vi "Check motor D2XX.vi"(8 "error in (no error)":errorcluster, 11 "AISAS control in":refnum<class "AISAS motor.lvclass">) -> (0 "error out":errorcluster, 2 "Motor Ok":bool, 3 "AISAS control out":refnum<class "AISAS motor.lvclass">)   [LabVIEW 2014, in "AISAS motor.lvclass"]
uses:
  AISAS motor.lvclass
  Controls/motor.ctl
  AISAS motor.lvclass/AISAS motor.ctl
panel:
  out "Motor":T1
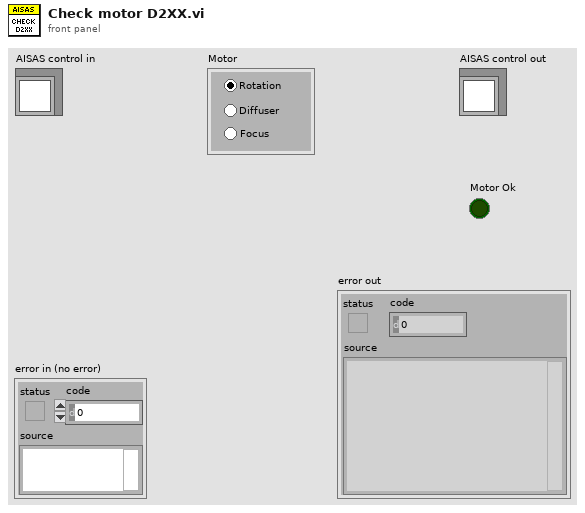
[diagram p1: front panel]
types:
  T1 = typedef "motor.ctl" = enum32{"Rotation", "Diffuser ", "Focus"}
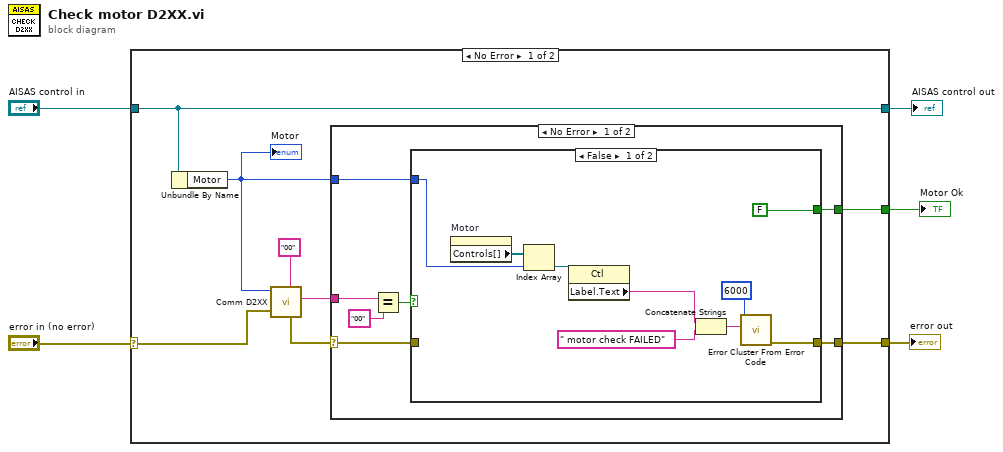
[diagram p0: block diagram]
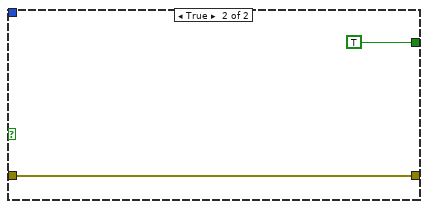
[diagram p2: hidden frame]
diagram:
  n1 = case shown="No Error" "error in (no error)" {
    selector: "error in (no error)" -> [w12 w34]
    tunnel: [w8 w34] -> w4
    tunnel: [w11 w33] -> w2
    tunnel: "AISAS control in" -> [w11 w33]
    tunnel: [w7 _] -> w1
    frame No Error {
      n2 = Unbundle By Name(w11) -> ("Motor"=w6:T1)
      "Motor" <- w6
      n3 = call "Comm D2XX.vi"("Motion Code"="00", "error in (no error)"=w12, "Motor"=w6) -> ("Read Buffer Out"=w9:string, "error out"=w10:errorcluster)  [unwired: 5 in, 2 out]
      n4 = case shown="No Error" w10 {
        selector: w10 -> [w18 w32]
        tunnel: w9 -> [w20 _]
        tunnel: w6 -> [w16 _]
        tunnel: [w15 w32] -> w8
        tunnel: [w14 _] -> w7
        frame No Error {
          n5 = Equal?(x=w20, y="00" ("Motion Code")) -> (x = y?=w17:bool)
          n6 = case shown="False" w17 {
            tunnel: w18 -> [_ w31]
            tunnel: w16 -> [w25 _]
            tunnel: [w28 w31] -> w15
            tunnel: [FALSE ("Motor Ok") TRUE ("Motor Ok")] -> w14
            frame False {
              n7 = property on="Motor" class="RadioBtnsControl (strict)"() -> ("Controls[]"=w26:refnum<vi>[])  [unwired: 2 in, 2 out]
              n8 = Index Array(array=w26, index=w25) -> (element=w24:refnum<vi>)
              n9 = property class="Ctl"(reference=w24) -> ("Label.Text"=w21:string)  [unwired: 1 in, 2 out]
              n10 = Concatenate Strings(w21, " motor check FAILED" ("error message (\"\")")) -> (w23:string)
              n11 = call <vilib>:"Error Cluster From Error Code.vi"("error message (\"\")"=w23, "error code (0)"=6000) -> ("error out"=w28:errorcluster)  [unwired: 7 in]
            }
            frame True {
            }
          }
        }
        frame Error {
        }
      }
    }
    frame Error {
    }
  }
  "error out" <- w4
  "AISAS control out" <- w2
  "Motor Ok" <- w1
